vi "Measurement_Server.vi"() -> ()   [LabVIEW 2021]
uses:
  Measurement_server/RPC Service/MeasurementService/MeasurementService.lvclass
  <vilib>/gRPC/LabVIEW gRPC Library/Shared/grpcId.ctl
  <vilib>/gRPC/LabVIEW gRPC Servicer/Servicer/Servicer.lvclass/Servicer.ctl
  Measurement_server/RPC Service/MeasurementService/MeasurementService.lvclass/MeasurementService.ctl
  Measurement_server/RPC Messages/measurement_DataPoint.ctl
  Measurement_server/RPC Messages/measurement_StatusResponse.ctl
  Measurement_server/RPC Messages/measurement_DataResponse.ctl
  Measurement_server/RPC Messages/measurement_ProcessResponse.ctl
  <vilib>/numeric/Random Number (Range) U64.vi
  <vilib>/Analysis/baseanly.llb/Mean (DBL).vi
  <vilib>/numeric/sub_Random U32.vi
  <vilib>/gRPC/LabVIEW gRPC Servicer/Servicer/Servicer.lvclass
  Measurement_server/Measurement_server.lvlib
  <vilib>/Analysis/NI_AALBase.lvlib
  <vilib>/gRPC/LabVIEW gRPC Library/grpc-lvsupport-release.lvlib
panel:
  out "Server_Time":string
  out "Acquired_Data":dbl[](array[numeric])
  out "Average":dbl format="%0.2f"
  out "RMS":dbl
  out "Running?":bool
  out "Waveform Chart":dbl(graph)
  in  "Server Address":string="localhost:50051"
  out "Listening Port":i32
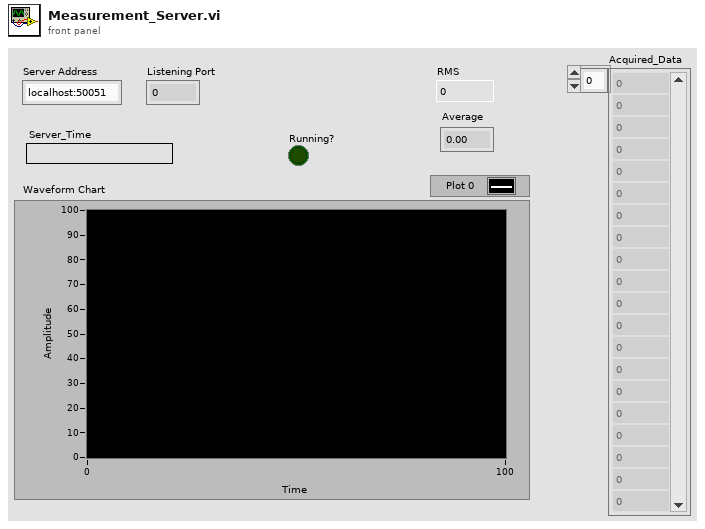
[diagram p1: front panel]
types:
  T1 = typedef "grpc-lvsupport-release.lvlib/grpcId.ctl" = u64
  T2 = cluster{"Running?":bool, "Stream_ID":T1, "Index":i32, "Wait":i32}
  T3 = typedef "Measurement_server.lvlib/MeasurementService.lvclass/Server gRPC UEs.ctl" = cluster{"MeasurementService GetStatus gRPC UE":refnum<user-event>, "MeasurementService AcquireSensorData gRPC UE":refnum<user-event>, "MeasurementService ProcessData gRPC UE":refnum<user-event>, "MeasurementService StreamSensorData gRPC UE":refnum<user-event>}
  T4 = typedef "Measurement_server.lvlib/measurement_DataPoint.ctl" = cluster{"value":dbl, "timestamp":i64}
  T5 = typedef "Measurement_server.lvlib/measurement_StatusResponse.ctl" = cluster{"server_time":string, "version":string}
  T6 = typedef "Measurement_server.lvlib/measurement_DataResponse.ctl" = cluster{"values":dbl[]}
  T7 = typedef "Measurement_server.lvlib/measurement_ProcessResponse.ctl" = cluster{"rms":dbl, "average":dbl}
  T8 = typedef "Measurement_server.lvlib/measurement_DataRequest.ctl" = cluster{"sample_count":i32}
  T9 = typedef "Measurement_server.lvlib/measurement_ProcessRequest.ctl" = cluster{"input_values":dbl[]}
  T10 = typedef "Measurement_server.lvlib/measurement_StreamRequest.ctl" = cluster{"interval_ms":i32}
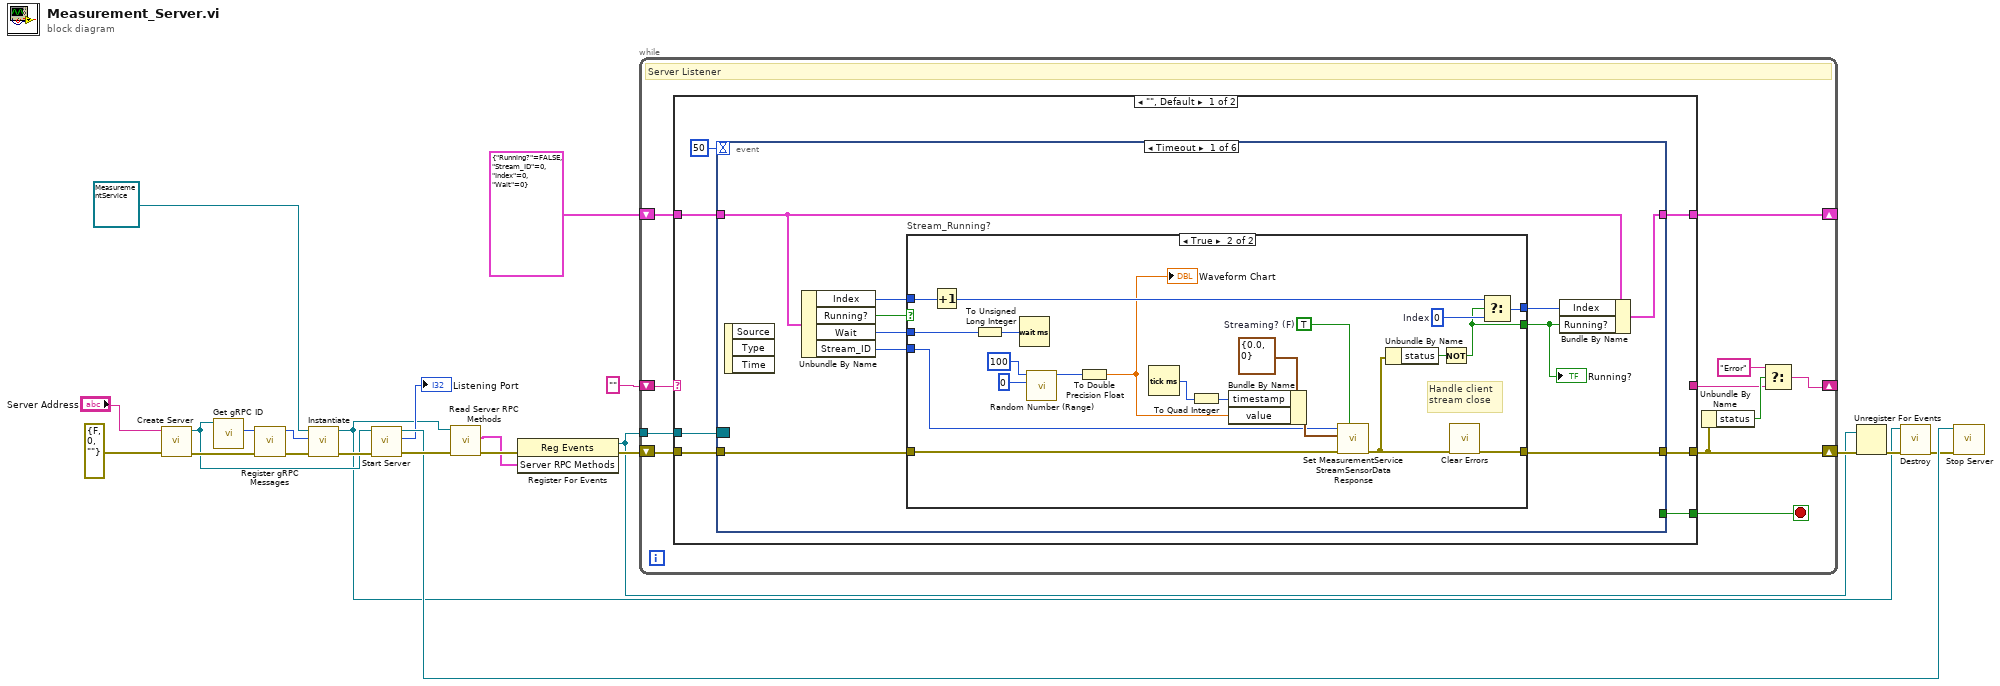
[diagram p0: block diagram]
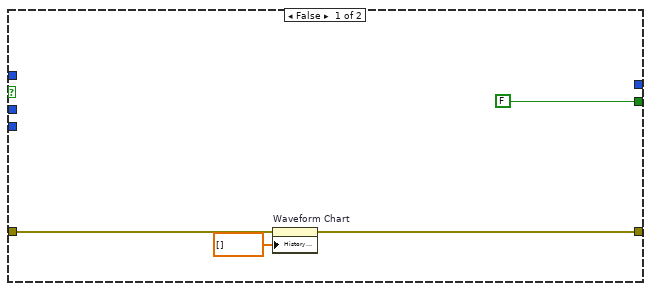
[diagram p2: hidden frame]
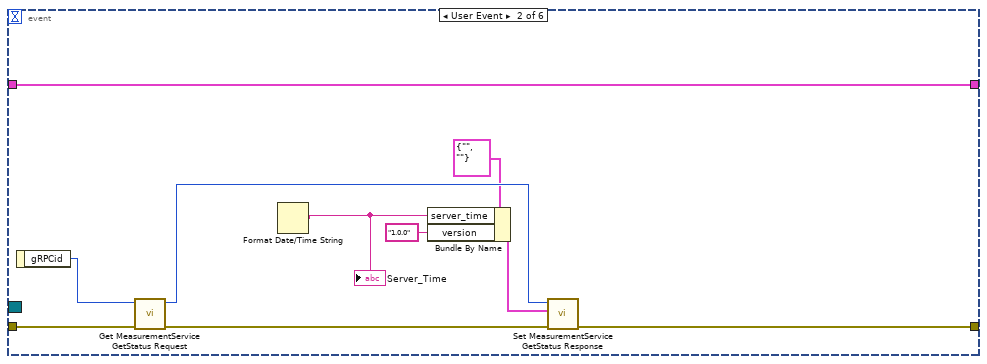
[diagram p3: hidden frame]
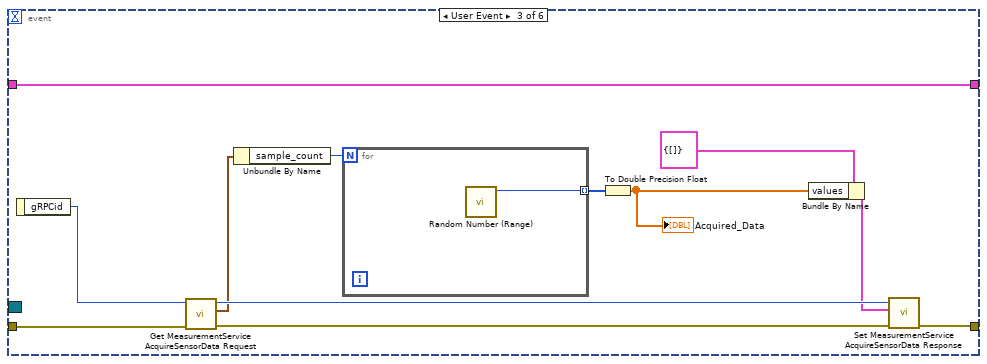
[diagram p4: hidden frame]
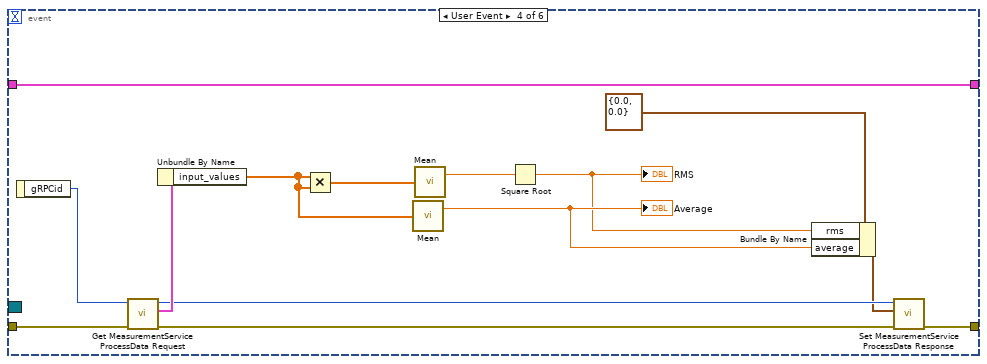
[diagram p5: hidden frame]
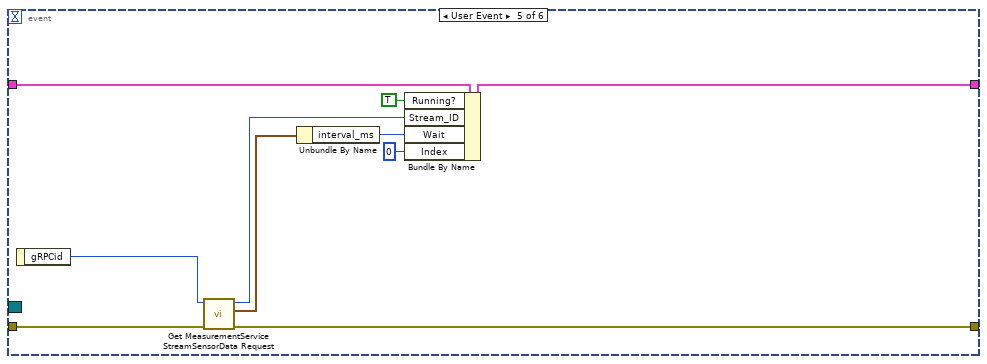
[diagram p6: hidden frame]
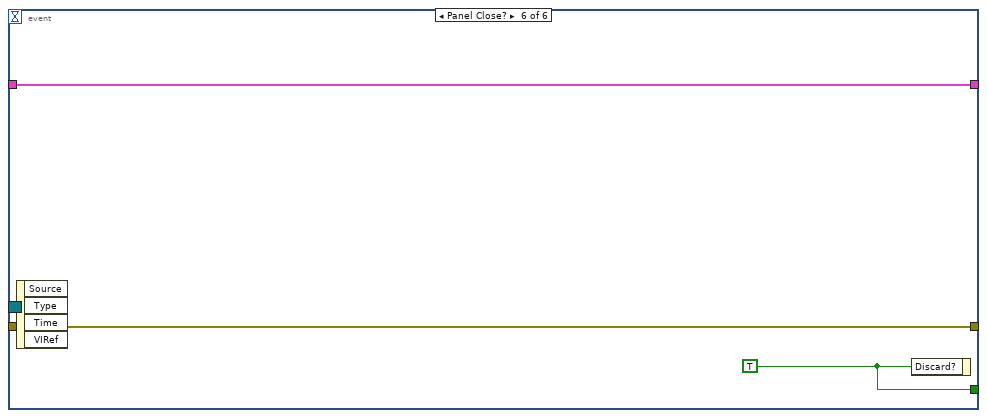
[diagram p7: hidden frame]
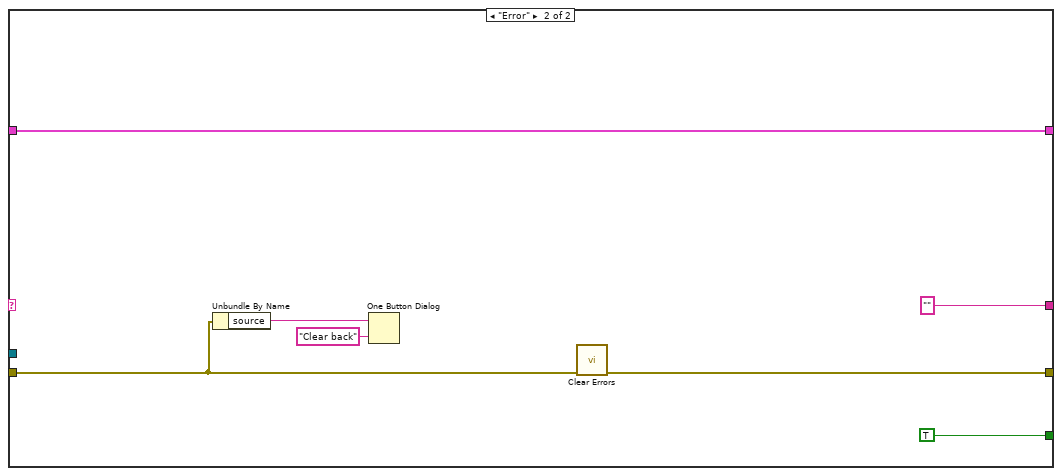
[diagram p8: hidden frame]
diagram:
  n1 = call <vilib>:"Create Server.vi"("error in"=errorcluster {"status"=FALSE, "code"=0, "source"=""} ("error in (no error)"), "Server Address"="Server Address") -> ("error out"=w14:errorcluster, "gRPC Server out"=w11:refnum<class "Servicer.lvclass">)  [unwired: 8 in]
  n2 = call <vilib>:"Get gRPC ID.vi"("OOP Server in"=w11) -> ("gRPC ID"=w15:T1)  [unwired: 9 in, 1 out]
  n3 = call "Register gRPC Messages.vi"("error in (no error)"=w14, "gRPC ID"=w15) -> ("error out"=w17:errorcluster, "gRPC ID Out"=w16:T1)  [unwired: 8 in]
  n4 = call-dynamic "Instantiate.vi"("error in"=w17, "gRPCid"=w16, "iService"=refnum<class "MeasurementService.lvclass"> refnum ("Measurement_server.lvlib:MeasurementService.lvclass")) -> ("error out"=w12:errorcluster, "iService"=w2:refnum<class "MeasurementService.lvclass">)  [unwired: 7 in]
  n5 = call <vilib>:"Start Server.vi"("error in"=w12, "gRPC Server in"=w11) -> ("error out"=w10:errorcluster, "Listening Port"=→"Listening Port":i32, "gRPC Server out"=w6:refnum<class "Servicer.lvclass">)  [unwired: 7 in]
  n6 = call "Read Server RPC Methods.vi"("error in (no error)"=w10, "SignalGeneratorService in"=w2) -> ("error out"=w9:errorcluster, "Server RPC Methods"=w7:T3)  [unwired: 7 in, 1 out]
  n7 = register-events(error in=w9, w7) -> (reference out=w19:refnum<event-registration>, error out=w21:errorcluster)  [unwired: 1 in]
  n8 = while {
    shift-right: [w30] -> w20
    shift-left: w21 -> [w32]
    shift-right: [w28] -> _
    shift-left: "" -> [w33]
    tunnel: w19 -> [w25]
    shift-right: [w23] -> _
    shift-left: T2 {"Running?"=FALSE, "Stream_ID"=0, "Index"=0, "Wait"=0} -> [w24]
    stop <- w31 stop-if-true
    # "Server Listener"
    n9 = case shown="\"\", Default" w33 {
      tunnel: w32 -> [w40 w131]
      tunnel: [w39 w132] -> w30
      tunnel: [_ ""] -> w27
      tunnel: [w38 TRUE ("Discard?")] -> w31
      tunnel: w25 -> [w36 _]
      tunnel: w24 -> [w35 w127]
      tunnel: [w34 w127] -> w23
      frame "", Default {
        n10 = event shown="[0] Timeout" {
          selector: w36 -> [_ _ _ _ _ _]
          dyn-events: _ -> [_ _ _ _ _ _]
          timeout: 50 -> [_ _ _ _ _ _]
          tunnel: w40 -> [w44 w85 w95 w110 w121 w125]
          tunnel: [w43 w82 w97 w112 w122 w125] -> w39
          tunnel: [_ _ _ _ _ w124] -> w38
          tunnel: w35 -> [w41 w76 w86 w99 w119 w123]
          tunnel: [w42 w76 w86 w99 w118 w123] -> w34
          event Timeout {
            n11 = event-data() -> ()  [unwired: 1 in, 3 out]
            n12 = Unbundle By Name(w41) -> ("Index"=w49:i32, "Running?"=w46:bool, "Wait"=w45:i32, "Stream_ID"=w50:T1)
            n13 = case "Stream_Running?" shown="True" w46 {
              tunnel: [w54 w60] -> w43
              tunnel: w44 -> [w53 w67]
              tunnel: w50 -> [_ w64]
              tunnel: w49 -> [_ w75]
              tunnel: [_ w73] -> w48
              tunnel: [FALSE w59] -> w47
              tunnel: w45 -> [_ w58]
              frame False {
                n14 = property on="Waveform Chart" class="WFChart (strict)"(error in=w53, "History Data"=dbl[] []) -> (error out=w54:errorcluster)  [unwired: 1 in, 1 out]
              }
              frame True {
                w63 = TRUE  # Streaming? (F)
                w72 = 0  # Index
                # "Handle client \nstream close"
                n15 = Increment(x=w75) -> (x+1=w74:i32)
                n16 = To Unsigned Long Integer(number=w58) -> (unsigned 32bit integer=w57:u32)
                n17 = Wait (ms)(milliseconds to wait=w57) -> ()  [unwired: 1 out]
                n18 = call-poly <vilib>:"Random Number (Range).vi"("lower bound (0)"=u64 0, "upper bound (100)"=u64 100) -> ("number"=w69:u64)  [unwired: 9 in]
                n19 = To Double Precision Float(number=w69) -> (double precision float=w68:dbl)
                "Waveform Chart" <- w68
                n20 = Tick Count (ms)() -> (millisecond timer value=w56:u32)
                n21 = To Quad Integer(1:w56) -> (0:w55:i64)
                n22 = Bundle By Name(cluster=T4 {"value"=0.0, "timestamp"=0} ("Message Data"), "timestamp"=w55, "value"=w68) -> (w65:T4)
                n23 = call "Set MeasurementService StreamSensorData Response.vi"("Streaming? (F)"=w63, "error in (no error)"=w67, "Message Data"=w65, "gRPCid in"=w64) -> ("error out"=w62:errorcluster)  [unwired: 7 in]
                n24 = Unbundle By Name(w62) -> ("status"=w61:bool)
                n25 = Not(x=w61) -> (.not. x?=w59:bool)
                n26 = call <vilib>:"Clear Errors.vi"("error in (no error)"=w62) -> ("error out"=w60:errorcluster)  [unwired: 5 in, 1 out]
                n27 = Select(t=w74, s=w59, f=w72) -> (s? t:f=w73:i32)
              }
            }
            "Running?" <- w47
            n28 = Bundle By Name(cluster=w41, "Index"=w48, "Running?"=w47) -> (w42:T2)
          }
          event User Event {
            n29 = event-data() -> ("gRPCid"=w84:T1)  [unwired: 1 in]
            n30 = call "Get MeasurementService GetStatus Request.vi"("error in (no error)"=w85, "gRPCid"=w84) -> ("error out"=w83:errorcluster, "gRPCid out"=w81:T1)  [unwired: 7 in, 1 out]
            n31 = Format Date/Time String() -> (date/time string=w77:string)  [unwired: 3 in]
            "Server_Time" <- w77
            n32 = Bundle By Name(cluster=T5 {"server_time"="", "version"=""} ("Message Data"), "server_time"=w77, "version"="1.0.0") -> (w79:T5)
            n33 = call "Set MeasurementService GetStatus Response.vi"("error in (no error)"=w83, "Message Data"=w79, "gRPCid in"=w81) -> ("error out"=w82:errorcluster)  [unwired: 8 in]
          }
          event User Event {
            n34 = event-data() -> ("gRPCid"=w94:T1)  [unwired: 1 in]
            n35 = call "Get MeasurementService AcquireSensorData Request.vi"("error in (no error)"=w95, "gRPCid"=w94) -> ("error out"=w96:errorcluster, "Message Data"=w92:T8, "gRPCid out"=w93:T1)  [unwired: 7 in]
            n36 = Unbundle By Name(w92) -> ("sample_count"=w91:i32)
            n37 = for {
              N: w91 -> [_]
              tunnel: [w98] -> w88 mode=indexing
              n38 = call-poly <vilib>:"Random Number (Range).vi"() -> ("number"=w98:u64)  [unwired: 11 in]
            }
            n39 = To Double Precision Float(number=w88) -> (double precision float=w87:dbl[])
            "Acquired_Data" <- w87
            n40 = Bundle By Name(cluster=T6 {"values"=[]} ("Message Data"), "values"=w87) -> (w89:T6)
            n41 = call "Set MeasurementService AcquireSensorData Response.vi"("error in (no error)"=w96, "Message Data"=w89, "gRPCid in"=w93) -> ("error out"=w97:errorcluster)  [unwired: 8 in]
          }
          event User Event {
            n42 = event-data() -> ("gRPCid"=w109:T1)  [unwired: 1 in]
            n43 = call "Get MeasurementService ProcessData Request.vi"("error in (no error)"=w110, "gRPCid"=w109) -> ("error out"=w111:errorcluster, "Message Data"=w108:T9, "gRPCid out"=w107:T1)  [unwired: 7 in]
            n44 = Unbundle By Name(w108) -> ("input_values"=w104:dbl[])
            n45 = Multiply(x=w104, y=w104) -> (x*y=w102:dbl[])
            n46 = call-poly <vilib>:"Mean.vi"("X"=w104) -> ("mean"=w103:dbl)  [unwired: 1 out]
            "Average" <- w103
            n47 = call-poly <vilib>:"Mean.vi"("X"=w102) -> ("mean"=w101:dbl)  [unwired: 1 out]
            n48 = Square Root(x=w101) -> (sqrt(x)=w100:dbl)
            "RMS" <- w100
            n49 = Bundle By Name(cluster=T7 {"rms"=0.0, "average"=0.0} ("Message Data"), "rms"=w100, "average"=w103) -> (w105:T7)
            n50 = call "Set MeasurementService ProcessData Response.vi"("error in (no error)"=w111, "Message Data"=w105, "gRPCid in"=w107) -> ("error out"=w112:errorcluster)  [unwired: 8 in]
          }
          event User Event {
            n51 = event-data() -> ("gRPCid"=w120:T1)  [unwired: 1 in]
            n52 = call "Get MeasurementService StreamSensorData Request.vi"("error in (no error)"=w121, "gRPCid"=w120) -> ("error out"=w122:errorcluster, "Message Data"=w115:T10, "gRPCid out"=w116:T1)  [unwired: 7 in]
            n53 = Unbundle By Name(w115) -> ("interval_ms"=w114:i32)
            n54 = Bundle By Name(cluster=w119, "Running?"=TRUE, "Stream_ID"=w116, "Wait"=w114, "Index"=0) -> (w118:T2)
          }
          event Panel Close? {
            w124 = TRUE ("Discard?")
            n55 = event-data() -> ()  [unwired: 1 in, 4 out]
            n56 = event-data("Discard?"=w124) -> ()  [unwired: 1 in, 1 out]
          }
        }
      }
      frame "Error" {
        n57 = Unbundle By Name(w131) -> ("source"=w129:string)
        n58 = One Button Dialog(message=w129, button name ("OK")="Clear back") -> ()  [unwired: 1 out]
        n59 = call <vilib>:"Clear Errors.vi"("error in (no error)"=w131) -> ("error out"=w132:errorcluster)  [unwired: 5 in, 1 out]
      }
    }
    n60 = Unbundle By Name(w30) -> ("status"=w29:bool)
    n61 = Select(t="Error", s=w29, f=w27) -> (s? t:f=w28:string)
  }
  n62 = Unregister For Events(event registration refnum=w19, error in=w20) -> (error out=w3:errorcluster)
  n63 = call-dynamic "Destroy.vi"("error in (no error)"=w3, "SignalGeneratorService in"=w2) -> ("error out"=w4:errorcluster)  [unwired: 8 in, 1 out]
  n64 = call <vilib>:"Stop Server.vi"("error in"=w4, "gRPC Server in"=w6) -> ()  [unwired: 9 in, 1 out]
